vi "ERIO Windows UI.vi"() -> ()   [LabVIEW 2017]
doc: "This is the primary host VI which acts as the conveyor simulation supervisory role. It updates the supervisory control variables from this UI to the SystemLink server, then retrieves process data updates from the various sources, and finally uses that data to update the supvisory HMI display window. \n\nDepending on which ones are enabled in this UI, the process data sources can be any of the following. \n- SystemLink server\n- AWS SQS Simple Queue Service\n- AWS SNS Simple Notification Service\n- AWS S3 Simple Storage bucket\n\nNOTE: This Windows supervisor program must be run first before the sbRIO process target to properly initialize process variables and enable correct simulation operation. \n\nORIGINAL CODE: \nBy: National Instruments\n NI LabVIEW RIO Evaluation Kit\n Code example \"5- Startup Application\"\n www.ni.com/embeddedsystems\n\nUPDATED CODE: Adds NI SystemLink and NI AWS LabVIEW Tookit functionality for demonstration. \nBy: James Tillett P.E.\n Endeavor Engineering Inc.\n www.endeavoreng.com"
uses:
  <vilib>/AWS Toolkit/Core/HTTP Request/Region.ctl
  Class EEISysLink/Controls/SL Tag Type.ctl
  LabVIEW/Controls/ERIO Supervisory Variables.ctl
  <vilib>/Utility/error.llb/DialogType.ctl
  Class EEISysLink/EEISysLink.lvclass
  LabVIEW/Controls/ERIO AWS Toolkit Variables.ctl
  <vilib>/AWS Toolkit/SQS/Queue/Queue.lvclass
  <vilib>/AWS Toolkit/SNS/Phone Number/Phone Number.lvclass
  <vilib>/AWS Toolkit/S3/Bucket/Bucket.lvclass
  LabVIEW/Controls/ERIO WIN State Variables.ctl
  LabVIEW/Controls/ERIO Worker Variables.ctl
  LabVIEW/Controls/ERIO Globals.vi
  <vilib>/AWS Toolkit/Core/HTTP Request/HTTP Request.lvclass
panel:
  out "Loop Iterations":i32
  in  "AWS S3 Bucket":string="mynicloud-demotest2"
  in  "AWS SQS Queue Name":string="mynicloud-demotest2"
  out "Alarm":bool
  in  "AWS SMS Phone Number":string="+15037066913"
  in  "AWS Region":T1=enum."us-west-2"
  in  "AWS Secret Key":string="1234567890abcdefghijklmnopqrstuvwxyz09876543221"
  in  "AWS Access Key":string="AKIAJETHPAD3QZJ2DKQBA"
  out "Stage Percent Complete":dbl(slide) scale=0.0..100.0
  out "Capture Update Time":timestamp
  out "Last Triggered Signal Capture":waveform(dbl)(graph)
  out "Operating State":string
  in  "Capture Signal":bool
  in  "Signal Alarm Threshold (volts)":dbl=4.2 format="%#_3g"
  in  "Signal Capture File Path":path=path "C:/ERIO Data Files"
  out "SQS Notifications (AWS)":string
  in  "Enable SystemLink Signal Capture":bool=TRUE
  in  "Enable S3 TDMS Signal Capture":bool
  in  "Enable SQS Notification":bool
  in  "Enable SNS Stage Notification":bool
  in  "Enable SNS Alarm Notification (SMS)":bool
  out "Stage 3":bool
  out "Stage 2":bool
  out "Stage 1":bool
  in  "Stop UI":bool
  out "Amplitude":dbl format="%#_3g"
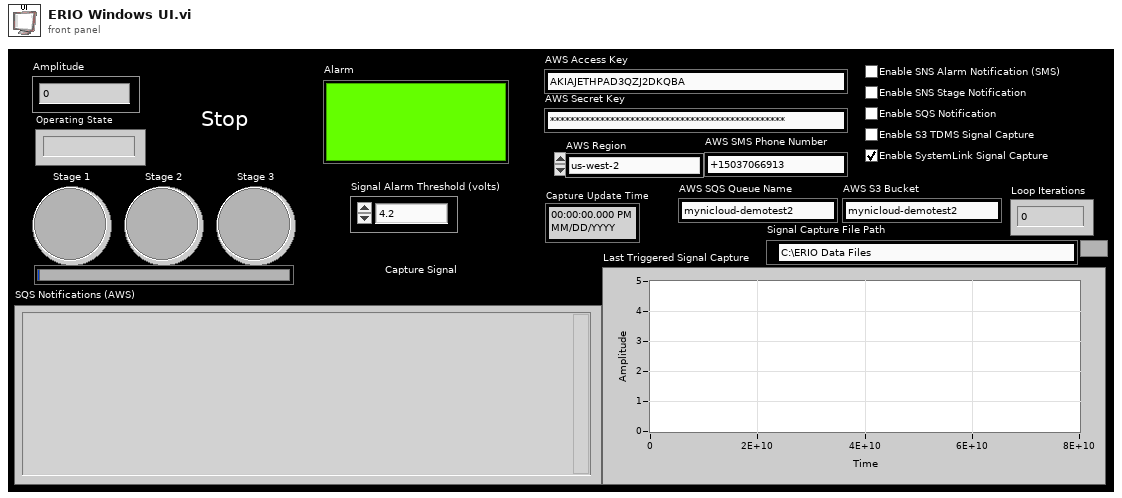
[diagram p1: front panel]
types:
  T1 = typedef "NI_AWS_Core.lvlib/HTTP Request.lvclass/Region.ctl" = enum16{"us-east-1", "us-east-2", "us-west-1", "us-west-2", "ap-northeast-1", "ap-northeast-2", "ap-southeast-1", "ap-southeast-2", "ca-central-1", "eu-central-1", "eu-west-1", "eu-west-2", "sa-east-1"}
  T2 = typedef "EEISysLink.lvclass/SL Tag Type.ctl" = enum16{"All", "Supervisor", "Worker"}
  T3 = typedef "ERIO Supervisory Variables.ctl" = cluster{"Alarm Threshold":dbl, "Shutdown":bool, "Enable SNS Alarm":bool, "Enable SNS Stage Notification":bool, "Enable SQS Notification":bool, "Enable S3 TDMS Signal Capture":bool, "Enable SystemLink Signal Capture":bool, "Capture Signal":bool, "Server Update":bool, "AWS Access Key":string, "AWS Secret Key":string, "Phone Number":string, "Region":T1, "AWS SQS Queue":string, "AWS S3 Bucket":string}
  T4 = typedef "ERIO WIN State Variables.ctl" = cluster{"Worker Variables":T5, "Notifications":string[], "New Capture":bool, "Last Signal Capture":waveform(dbl)}
  T5 = typedef "ERIO Worker Variables.ctl" = cluster{"Signal Amplitude":dbl, "State":string, "Stage Percent Complete":dbl, "Alarm State":bool, "Capture Available":bool}
  T6 = typedef "ERIO AWS Toolkit Variables.ctl" = cluster{"SQS Queue":refnum<class "Queue.lvclass">, "SNS Phone Number":refnum<class "Phone Number.lvclass">, "S3 Bucket":refnum<class "Bucket.lvclass">, "SQS Init?":bool, "S3 Init?":bool, "SNS Init?":bool}
  T7 = typedef "SL Tag Value.ctl" = cluster{"Value":variant, "Time Stamp":timestamp, "Tag Data Type":T8, "Name":string}
  T8 = typedef "EEISysLink.lvclass/SL Tag Data Type.ctl" = enum16{"Double", "Integer", "String", "Boolean", "Waveform"}
  T9 = typedef "EEISysLink.lvclass/SL Tag Properties.ctl" = cluster{"Class Data Type":T8, "Name":string, "Description":string, "Interpolation Method":T10, "Unit of Measure":T11, "Maximum Interpolation":string, "Role":T2}
  T10 = typedef "EEISysLink.lvclass/SL Tag Interpolation Method.ctl" = enum16{"linear", "pilinear", "step"}
  T11 = typedef "EEISysLink.lvclass/SL Tag Unit of Measure.ctl" = enum16{"no units", "Second", "Hour", "Minute", "Day", "Year", "Month", "Week", "Foot", "Yard", "Meter", "Centimeter", "Inch", "Mile", "Nautical Mile", "Miles per Hour", "Meters per second", "Square meter", "Cubic meter", "Cubic centimeter", "Cubic inch", "Liter", "Gallon", "Gallons dry US", "Gallon UK", "Percent", "Revolutions per minute", "Revolution", "Degree angle", "Astronomical Unit", "Atom", "Atomic mass", "Bar", "Byte", "C (speed of light)", "Curie", "Decibel", "Electron Volt", "Ounce", "Knot", "G", "Grade", "Are", "Hectare", "Faraday", "Franklin", "Gilbert", "Erg", "Lambert", "Maxwell", "Gauss", "Electron mass", "Kilogram force", "Pound force", "Rad", "Centiradian", "Sphere", "Mach", "Fluid Ounces", "Fluid Ounces UK", "Fahrenheit", "Celsius", "Kelvin", "Rankine", "Gram", "Kilogram", "Pound", "Short/US Ton", "Long/UK ton", "Metric ton", "Mole", "Pounds per square inch", "Inches water column", "Torr", "Millitorr", "Millimeter mercury", "Inches mercury", "Bar (2)", "Atmosphere", "Pascal", "Watt", "kiloWatt", "Horsepower", "Kilowatt Hour", "British thermal units", "Millions of BTU", "Ampere", "Candela", "Radian", "Steradian", "Bit", "Hertz", "Newton", "Joule", "Coulomb", "Volt", "Farad", "Ohm", "Siemens", "Weber", "Tesla", "Henry", "Lumen", "Lux", "Becqueral", "Gray", "Sievert", "Katal", "Angstrom", "Light Year", "Parsec", "Point", "Pixel", "Dyne", "Kilogram force (2)", "Pound force (2)", "Rem", "Rutherford", "Roentgen"}
  T12 = typedef "DialogType.ctl" = u16
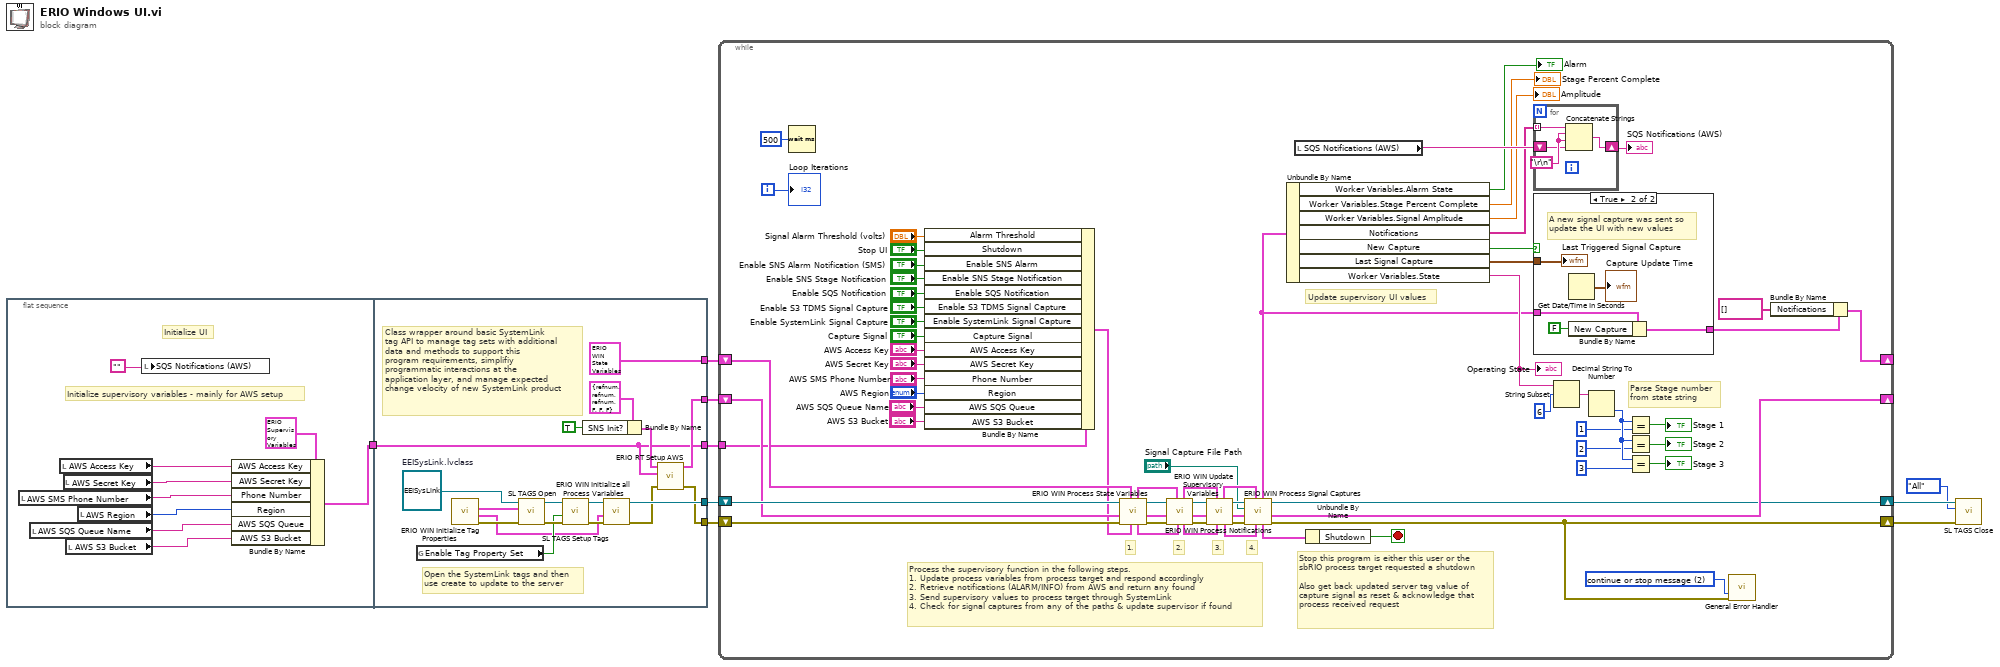
[diagram p0: block diagram]
diagram:
  n1 = flat-sequence {
    tunnel: [w12] -> w2
    tunnel: [w29] -> w6
    tunnel: [w19] -> w5
    tunnel: [T4 {"Worker Variables"={"Signal Amplitude"=0.0, "State"="", "Stage Percent Complete"=0.0, "Alarm State"=FALSE, "Capture Available"=FALSE}, "Notifications"=[], "New Capture"=FALSE, "Last Signal Capture"={"t0"=timestamp(0 s since 1904-01-01), "dt"=1.0, "Y"=[]}} ("Win State Variables")] -> w4
    tunnel: [w22] -> w3
    tunnel: w2 -> [w21]
    tunnel: [w21] -> w1
    frame #0 {
      # "Initialize supervisory variables - mainly for AWS setup"
      # "Initialize UI"
      n2 = local read "AWS SMS Phone Number"() -> (w15:string)
      n3 = local read "AWS SQS Queue Name"() -> (w17:string)
      n4 = local read "AWS Access Key"() -> (w13:string)
      n5 = local read "AWS Secret Key"() -> (w14:string)
      n6 = local read "AWS S3 Bucket"() -> (w18:string)
      n7 = local read "AWS Region"() -> (w16:T1)
      n8 = local write "SQS Notifications (AWS)"("") -> ()
      n9 = Bundle By Name(cluster=T3 {"Alarm Threshold"=0.0, "Shutdown"=FALSE, "Enable SNS Alarm"=FALSE, "Enable SNS Stage Notification"=FALSE, "Enable SQS Notification"=FALSE, "Enable S3 TDMS Signal Capture"=FALSE, "Enable SystemLink Signal Capture"=FALSE, "Capture Signal"=FALSE, "Server Update"=FALSE, "AWS Access Key"="AKIAINLDO2Y2PDFEWDOQ", "AWS Secret Key"="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", "Phone Number"="+15037066913", "Region"=enum."us-west-2", "AWS SQS Queue"="+15037066913", "AWS S3 Bucket"="+15037066913"} ("Supervisory Variables"), "AWS Access Key"=w13, "AWS Secret Key"=w14, "Phone Number"=w15, "Region"=w16, "AWS SQS Queue"=w17, "AWS S3 Bucket"=w18) -> (w12:T3)
    }
    frame #1 {
      w36 = refnum<class "EEISysLink.lvclass"> refnum  # EEISysLink.lvclass
      # "Class wrapper around basic SystemLink\ntag API to manage tag sets with additional\ndata and methods to support this \nprogram requirements, simplifiy\nprogrammatic interactions at the \napplication layer, and manage expected\nchange velocity of new SystemLink product"
      # "Open the SystemLink tags and then\nuse create to update to the server"
      n10 = global read "ERIO Globals.vi" "Enable Tag Property Set"() -> (w32:bool)
      n11 = call "ERIO WIN Initialize Tag Properties.vi"() -> ("error out"=w33:errorcluster, "Tag Update Values"=w27:T7[], "Tag Properties"=w28:T9[])  [unwired: 9 in]
      n12 = call-dynamic "SL TAGS Open.vi"("error in (no error)"=w33, "Tag Properties"=w28, "EEISysLink in"=w36) -> ("error out"=w35:errorcluster, "EEISysLink out"=w34:refnum<class "EEISysLink.lvclass">)  [unwired: 7 in]
      n13 = call-dynamic "SL TAGS Setup Tags.vi"("error in (no error)"=w35, "Set  Properties? (F)"=w32, "EEISysLink in"=w34) -> ("error out"=w30:errorcluster, "EEISysLink out"=w31:refnum<class "EEISysLink.lvclass">)  [unwired: 7 in]
      n14 = Bundle By Name(cluster=T6 {"SQS Queue"=refnum, "SNS Phone Number"=refnum, "S3 Bucket"=refnum, "SQS Init?"=FALSE, "S3 Init?"=FALSE, "SNS Init?"=FALSE} ("AWS Variables In"), "SNS Init?"=TRUE) -> (w23:T6)
      n15 = call "ERIO WIN Initialize all Process Variables.vi"("error in (no error)"=w30, "Tag Update Values"=w27, "EEISysLink.lvclass In"=w31) -> ("error out"=w20:errorcluster, "EEISysLink.lvclass Out"=w29:refnum<class "EEISysLink.lvclass">)  [unwired: 7 in]
      n16 = call "ERIO RT Setup AWS.vi"("error in (no error)"=w20, "Supervisory Variables"=w21, "AWS Variables In"=w23) -> ("error out"=w19:errorcluster, "AWS Variables Out"=w22:T6)  [unwired: 7 in]
    }
  }
  n17 = while {
    shift-right: [w54] -> w9
    shift-left: w6 -> [w92]
    shift-right: [w56] -> w8
    shift-left: w5 -> [w91]
    shift-right: [w55] -> _
    shift-left: w3 -> [w80]
    shift-right: [w39] -> _
    shift-left: w4 -> [w74]
    tunnel: w1 -> [w42]
    i -> [w37]
    stop <- w69 stop-if-true
    w67 = T12 2 items=["no dialog", "OK message", "continue or stop message", "OK message + warnings", "continue/stop + warnings"] ("type of dialog (OK msg:1)")
    # "4."
    # "3."
    # "2."
    # "1."
    # "Process the supervisory function in the following steps. \n1. Update process variables from process target and respond accordingly\n2. Retrieve notifications (ALARM/INFO) from AWS and return any found\n3. Send supervisory values to process target through SystemLink\n4. Check for signal captures from any of the paths & update supervisor if found"
    # "Update supervisory UI values"
    # "Stop this program is either this user or the\nsbRIO process target requested a shutdown\n\nAlso get back updated server tag value of\ncapture signal as reset & acknowledge that\nprocess received request"
    # "Parse Stage number\nfrom state string"
    n18 = Wait (ms)(milliseconds to wait=u32 500) -> ()  [unwired: 1 out]
    n19 = Bundle By Name(cluster=w42, "Alarm Threshold"="Signal Alarm Threshold (volts)", "Shutdown"="Stop UI", "Enable SNS Alarm"="Enable SNS Alarm Notification (SMS)", "Enable SNS Stage Notification"="Enable SNS Stage Notification", "Enable SQS Notification"="Enable SQS Notification", "Enable S3 TDMS Signal Capture"="Enable S3 TDMS Signal Capture", "Enable SystemLink Signal Capture"="Enable SystemLink Signal Capture", "Capture Signal"="Capture Signal", "AWS Access Key"="AWS Access Key", "AWS Secret Key"="AWS Secret Key", "Phone Number"="AWS SMS Phone Number", "Region"="AWS Region", "AWS SQS Queue"="AWS SQS Queue Name", "AWS S3 Bucket"="AWS S3 Bucket") -> (w65:T3)
    n20 = call "ERIO WIN Process State Variables.vi"("Supervisory Variables In"=w65, "WIN State In"=w74, "error in (no error)"=w91, "AWS Variables In"=w80, "EEISysLink.lvclass In"=w92) -> ("error out"=w89:errorcluster, "AWS Variables Out"=w79:T6, "EEISysLink.lvclass Out"=w90:refnum<class "EEISysLink.lvclass">, "Supervisory Variables Out"=w78:T3, "WIN State Out"=w77:T4)  [unwired: 2 in]
    n21 = call "ERIO WIN Process Notifications.vi"("Supervisory Variables In"=w78, "WIN Variables In"=w77, "error in (no error)"=w89, "AWS Variables In"=w79, "EEISysLink.lvclass In"=w90) -> ("error out"=w51:errorcluster, "AWS Variables Out"=w52:T6, "EEISysLink.lvclass Out"=w53:refnum<class "EEISysLink.lvclass">, "Supervisory Variables Out"=w50:T3, "WIN Variables Out"=w49:T4)  [unwired: 2 in]
    n22 = call "ERIO WIN Update Supervisory Variables.vi"("Supervisory Variables In"=w50, "WIN State In"=w49, "error in (no error)"=w51, "AWS Variables In"=w52, "EEISysLink.lvclass In"=w53) -> ("error out"=w57:errorcluster, "AWS Variables Out"=w58:T6, "EEISysLink.lvclass Out"=w59:refnum<class "EEISysLink.lvclass">, "Supervisory Variables Out"=w48:T3, "WIN State Out"=w45:T4)  [unwired: 2 in]
    n23 = call "ERIO WIN Process Signal Captures.vi"("Supervisory Variables In"=w48, "WIN Variables In"=w45, "error in (no error)"=w57, "AWS Variables In"=w58, "Signal Capture File Path"="Signal Capture File Path", "EEISysLink.lvclass In"=w59) -> ("error out"=w56:errorcluster, "AWS Variables Out"=w55:T6, "EEISysLink.lvclass Out"=w54:refnum<class "EEISysLink.lvclass">, "Supervisory Variables Out"=w47:T3, "WIN Variables Out"=w46:T4)  [unwired: 1 in]
    n24 = Unbundle By Name(w46) -> ("Worker Variables.Alarm State"=→"Alarm":bool, "Worker Variables.Stage Percent Complete"=→"Stage Percent Complete":dbl, "Worker Variables.Signal Amplitude"=→"Amplitude":dbl, "Notifications"=w71:string[], "New Capture"=w73:bool, "Last Signal Capture"=w72:waveform(dbl), "Worker Variables.State"=w70:string)
    "Operating State" <- w70
    n25 = local read "SQS Notifications (AWS)"() -> (w76:string)
    n26 = Unbundle By Name(w47) -> ("Shutdown"=w69:bool)
    n27 = for {
      tunnel: w71 -> [w112] mode=indexing
      shift-right: [w111] -> w75
      shift-left: w76 -> [w109]
      w110 = "\r\n"
      n28 = Concatenate Strings(w112, w110, w110, w109) -> (w111:string)
    }
    "SQS Notifications (AWS)" <- w75
    n29 = case shown="True" w73 {
      tunnel: w72 -> [_ w107]
      tunnel: w46 -> [w103 w106]
      tunnel: [w103 w104] -> w41
      frame False {
      }
      frame True {
        # "A new signal capture was sent so\nupdate the UI with new values"
        n30 = Get Date/Time In Seconds() -> (seconds since 1Jan1904=→"Capture Update Time":timestamp)
        n31 = Bundle By Name(cluster=w106, "New Capture"=FALSE) -> (w104:T4)
        "Last Triggered Signal Capture" <- w107
      }
    }
    n32 = String Subset(string=w70, offset (0)=6) -> (substring=w97:string)  [unwired: 1 in]
    n33 = Decimal String To Number(string=w97) -> (number=w96:i32)  [unwired: 2 in, 1 out]
    n34 = Equal?(x=w96, y=1 ("offset (0)")) -> (x = y?=→"Stage 1":bool)
    n35 = Equal?(x=w96, y=2 ("offset (0)")) -> (x = y?=→"Stage 2":bool)
    n36 = Equal?(x=w96, y=3 ("offset (0)")) -> (x = y?=→"Stage 3":bool)
    n37 = call <vilib>:"General Error Handler.vi"("type of dialog (OK msg:1)"=w67, "error in (no error)"=w56) -> ()  [unwired: 9 in, 5 out]
    n38 = Bundle By Name(cluster=w41, "Notifications"=string[] []) -> (w39:T4)
    "Loop Iterations" <- w37
  }
  n39 = call-dynamic "SL TAGS Close.vi"("error in (no error)"=w8, "Tag Type"=SL_Tag_Type."All", "EEISysLink in"=w9) -> ()  [unwired: 7 in, 2 out]
